vi "SSH_Init.vi"(8 "error in (no error)":errorcluster, 10 "Raspberry Pi":T2={"IP Address"="raspberrypi.local", "Username"="pi", "password"="raspberry"}, 11 "Python in":T1) -> (0 "error out":errorcluster, 1 "Console out":string, 3 "Python out":T1)   [LabVIEW 2021]
uses:
  PythonCtrl.ctl
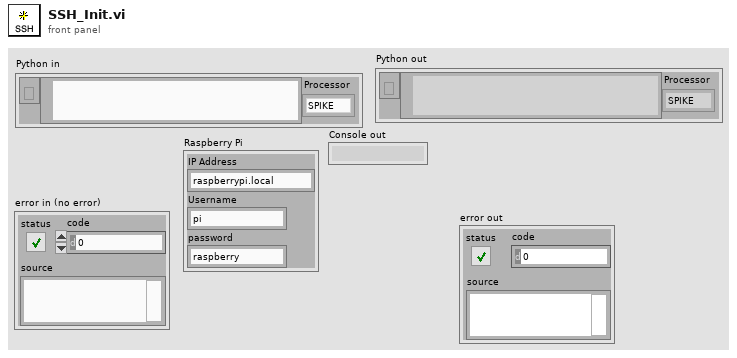
[diagram p1: front panel]
types:
  T1 = typedef "PythonCtrl.ctl" = cluster{"session":refnum<k35>, "PyPath":path, "Processor":enum16{"SPIKE", "Pi", "Pi_ssh"}}
  T2 = cluster{"IP Address":string, "Username":string, "password":string}
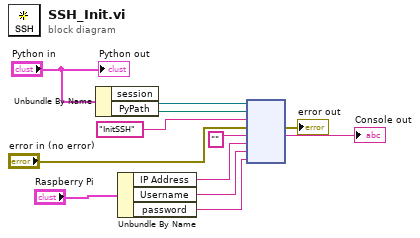
[diagram p0: block diagram]
diagram:
  n1 = Unbundle By Name("Python in") -> ("session"=w4:refnum<k35>, "PyPath"=w3:path)
  n2 = Unbundle By Name("Raspberry Pi") -> ("IP Address"=w10:string, "Username"=w9:string, "password"=w8:string)
  n3 = node(w4, w3, "InitSSH" ("function name"), "error in (no error)", "" ("function name"), w10, w9, w8) -> (→"error out":errorcluster, →"Console out":string)  [unwired: 3 in, 3 out]
  "Python out" <- "Python in"
